vi "PiezoSlew.vi"(4 "To":dbl, 5 "From":dbl, 6 "error in (no error)":errorcluster) -> (0 "error out":errorcluster)   [LabVIEW 2009]
uses:
  <vilib>/DAQmx/write.llb/DAQmx Write (Analog Wfm 1Chan NSamp).vi
  <vilib>/DAQmx/configure/timing.llb/DAQmx Timing (Use Waveform).vi
  <vilib>/DAQmx/create/channels.llb/DAQmx Create Channel (AO-Voltage-Basic).vi
  <vilib>/measure/NI_MABase.lvlib
panel:
  out "Graphe":waveform(dbl)(graph)
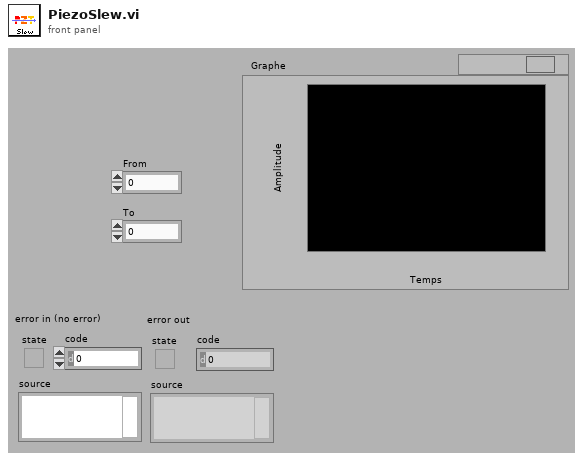
[diagram p1: front panel]
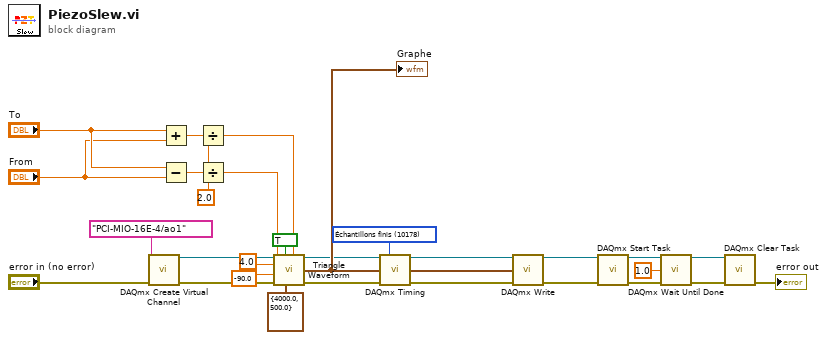
[diagram p0: block diagram]
diagram:
  w13 = 10178 items=["Échantillons finis"=10178, "Échantillons continus"=10123, "Point par point avec cadencement matériel"=12522] ("sample mode")
  w25 = 2.0 ("y")
  n1 = call-poly <vilib>:"DAQmx Create Virtual Channel.vi"("physical channels"=tag "PCI-MIO-16E-4/ao1", "error in"="error in (no error)") -> ("task out"=w2:refnum<k21>, "error out"=w3:errorcluster)  [unwired: 12 in]
  n2 = Add(x="To", y="From") -> (x+y=w26:dbl)
  n3 = Subtract(x="To", y="From") -> (x-y=w27:dbl)
  n4 = Divide(x=w26, y=w25) -> (x/y=w22:dbl)
  n5 = Divide(x=w27, y=w25) -> (x/y=w21:dbl)
  n6 = call <vilib>:"Triangle Waveform.vi"("offset"=w22, "sampling info"=cluster{"Fs":dbl, "#s":dbl} {"Fs"=4000.0, "#s"=500.0}, "reset signal"=TRUE, "error in (no error)"=w3, "phase"=-90.0, "amplitude"=w21, "frequency"=4.0) -> ("error out"=w17:errorcluster, "signal out"=w14:waveform(dbl))  [unwired: 3 in]
  "Graphe" <- w14
  n7 = call-poly <vilib>:"DAQmx Timing.vi"("task/channels in"=w2, "sample mode"=w13, "waveform"=w14, "error in"=w17) -> ("task out"=w15:refnum<k21>, "error out"=w16:errorcluster)  [unwired: 10 in]
  n8 = call-poly <vilib>:"DAQmx Write.vi"("task/channels in"=w15, "data"=w14, "error in"=w16) -> ("task out"=w11:refnum<k21>, "error out"=w12:errorcluster)  [unwired: 10 in, 1 out]
  n9 = call <vilib>:"DAQmx Start Task.vi"("task/channels in"=w11, "error in"=w12) -> ("task out"=w9:refnum<k21>, "error out"=w10:errorcluster)  [unwired: 12 in]
  n10 = call <vilib>:"DAQmx Wait Until Done.vi"("task/channels in"=w9, "timeout (sec)"=1.0, "error in"=w10) -> ("task out"=w8:refnum<k21>, "error out"=w7:errorcluster)  [unwired: 11 in]
  n11 = call <vilib>:"DAQmx Clear Task.vi"("task in"=w8, "error in"=w7) -> ("error out"=→"error out":errorcluster)  [unwired: 13 in]
